vi "Vm_and_g1g2g3_Wrapper.vi"(0 "Path Array":string[](array[string])=["C:\\CuspControl\\GPIB and Network\\RGSBias.txt", "6723"], 1 "Input Values":dbl[](array[numeric])=[88.0, 1.0, 2.0, 3.0]) -> ()   [LabVIEW 2018]
uses:
  <vilib>/Analysis/1siggen.llb/Ramp Pattern by Samples.vi
  <vilib>/DAQmx/write.llb/DAQmx Write (Analog 1D DBL 1Chan NSamp).vi
  <vilib>/DAQmx/create/channels.llb/DAQmx Create Channel (AO-Voltage-Basic).vi
  <vilib>/DAQmx/configure/timing.llb/DAQmx Timing (Sample Clock).vi
  <vilib>/DAQmx/miscellaneous.llb/DAQmx Fill In Error Info.vi
  <vilib>/Analysis/NI_AALBase.lvlib
panel:
  out "Vout, gain, offset":dbl[][](array[numeric])=[[0.0, 161.0, -0.006], [70.5, 161.0, -0.006], [79.5, 161.0, -0.006], [83.0, 161.0, -0.006], [0.0, 0.0, 0.0], [0.0, 0.0, 0.0], [0.0, 0.0, 0.0], [0.0, 0.0, 0.0], [0.0, 0.0, 0.0]]
  out "Output Values":dbl[](array[numeric])=[88.0, 1.0, 2.0, 3.0]
  out "pathName":path=path "C:/CuspControl/GPIB and Network/RGSBias.txt"
  in  "rate":dbl=1000.0 format="%0.2f"
  in  "samples":i32=128
  out "Start Values":dbl[](array[numeric])=[-3.7267080745341614e-05, 0.4378509316770186, 0.4937515527950311, 0.5154906832298136]
  out "End Values":dbl[](array[numeric])=[0.5465465838509317, 0.0061739130434782605, 0.012385093167701863, 0.018596273291925466]
  out "Enable":bool[](array[boolean])=[TRUE, TRUE, TRUE, TRUE]
  out "Time (s)":dbl=0.5339438999999402
  out "Device names":string[](array[string])=["Dev8/ao4", "Dev8/ao1", "Dev8/ao2", "Dev8/ao3"]
  out "error out":errorcluster
  # "RGS Bias Dev5/ao4"
  # "2021-07-27 EDH\nwtf Andi it's not dev5\nseems to be dev8\nin any case, is PXI 6723"
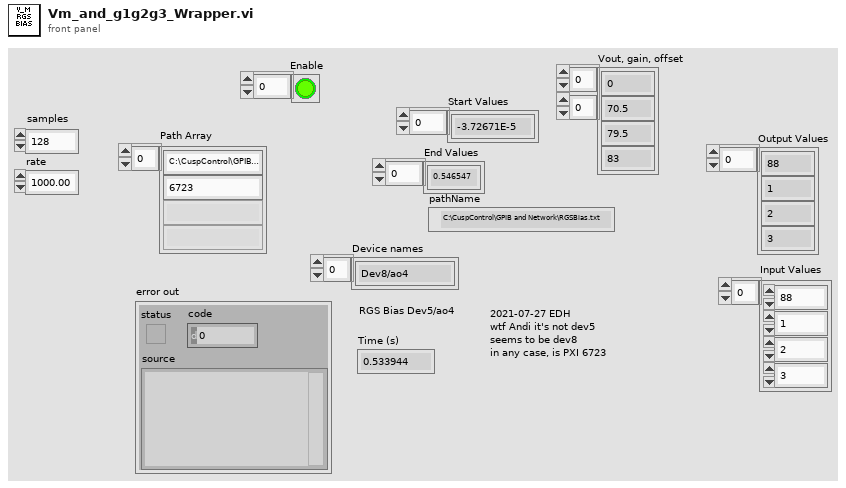
[diagram p1: front panel]
types:
  T1 = enum16{"open", "replace", "create", "open or create", "replace or create", "replace or create with confirmation"}
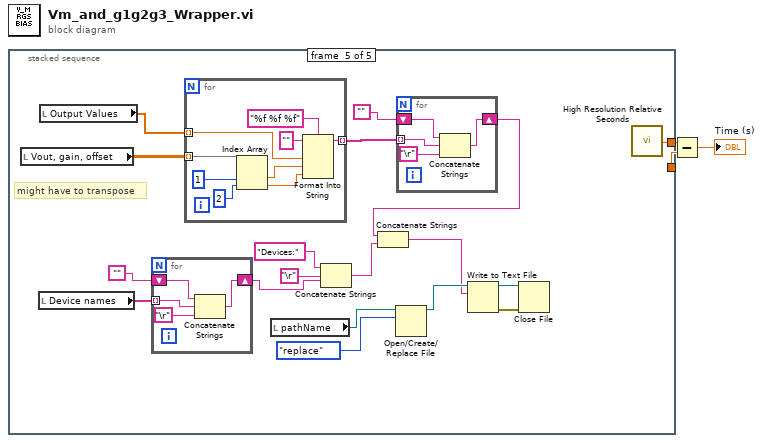
[diagram p0: block diagram]
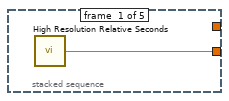
[diagram p2: hidden frame]
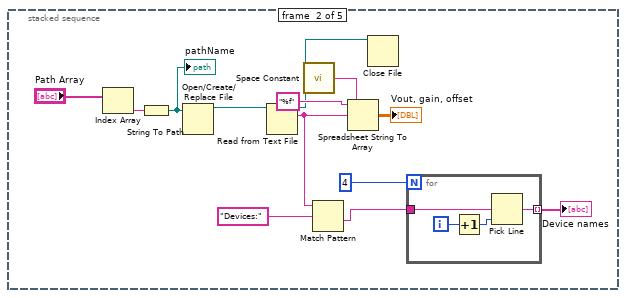
[diagram p3: hidden frame]
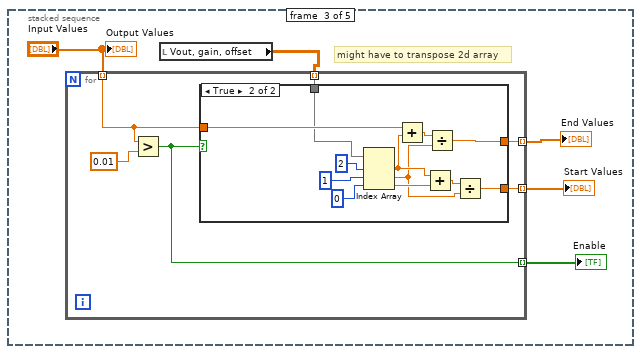
[diagram p4: hidden frame]
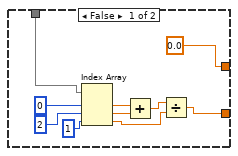
[diagram p5: hidden frame]
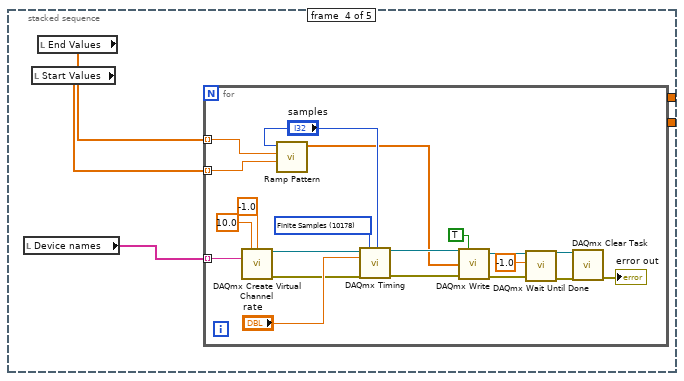
[diagram p6: hidden frame]
diagram:
  n1 = stacked-sequence {
    tunnel: [w4 _ _ _ _] -> w2
    tunnel: [_ _ _ _ w95] -> w3
    frame #0 {
      n2 = call <vilib>:"High Resolution Relative Seconds.vi"() -> ("relative seconds"=w4:dbl)
    }
    frame #1 {
      n3 = Index Array(array="Path Array") -> (element=w16:string)  [unwired: 1 in]
      n4 = String To Path(string=w16) -> (path=w7:path)
      "pathName" <- w7
      n5 = Open/Create/Replace File(file path (use dialog)=w7) -> (refnum out=w8:refnum<file>)  [unwired: 5 in, 2 out]
      n6 = Read from Text File(file (use dialog)=w8) -> (refnum out=w6:refnum<file>, text=w13:string)  [unwired: 3 in, 2 out]
      n7 = call <vilib>:"Space Constant.vi"() -> ("String"=w14:string)
      n8 = Match Pattern(string=w13, regular expression="Devices:") -> (after substring=w11:string)  [unwired: 1 in, 3 out]
      n9 = Spreadsheet String To Array(delimiter (Tab)=w14, format string="%f", spreadsheet string=w13) -> (array=→"Vout, gain, offset":dbl[][])  [unwired: 1 in]
      n10 = Close File(refnum=w6) -> ()  [unwired: 1 in, 2 out]
      n11 = for {
        N: 4 -> [_]
        tunnel: w11 -> [w19]
        tunnel: [w18] -> w9 mode=indexing
        i -> [w21]
        n12 = Increment(x=w21) -> (x+1=w20:i32)
        n13 = Pick Line(multi-line string=w19, line index=w20) -> (output string=w18:string)  [unwired: 1 in]
      }
      "Device names" <- w9
    }
    frame #2 {
      # "might have to transpose 2d array"
      n14 = local read "Vout, gain, offset"() -> (w22:dbl[][])
      n15 = for {
        tunnel: [w31] -> w26 mode=indexing
        tunnel: [w30] -> w25 mode=indexing
        tunnel: [w29] -> w24 mode=indexing
        tunnel: "Input Values" -> [w28] mode=indexing
        tunnel: w22 -> [w27] mode=indexing
        n16 = Greater?(x=w28, y=0.01) -> (0:w31:bool)
        n17 = case shown="True" w31 {
          tunnel: [0.0 w51] -> w30
          tunnel: w28 -> [_ w50]
          tunnel: [w39 w47] -> w29
          tunnel: w27 -> [w33 w43]
          frame False {
            n18 = Index Array(array=w33, index #1=0 ("index"), index #2=2 ("index"), index #3=1 ("index")) -> (element #1=w36:dbl, element #2=w35:dbl, element #3=w34:dbl)
            n19 = Add(x=w36, y=w35) -> (x+y=w41:dbl)
            n20 = Divide(x=w41, y=w34) -> (x/y=w39:dbl)
          }
          frame True {
            n21 = Index Array(array=w43, index #1=2 ("index"), index #2=1 ("index"), index #3=0 ("index")) -> (element #1=w45:dbl, element #2=w44:dbl, element #3=w46:dbl)
            n22 = Add(x=w50, y=w45) -> (x+y=w54:dbl)
            n23 = Add(x=w45, y=w46) -> (x+y=w48:dbl)
            n24 = Divide(x=w54, y=w44) -> (x/y=w51:dbl)
            n25 = Divide(x=w48, y=w44) -> (x/y=w47:dbl)
          }
        }
      }
      "Enable" <- w26
      "End Values" <- w25
      "Start Values" <- w24
      "Output Values" <- "Input Values"
    }
    frame #3 {
      n26 = local read "Device names"() -> (w55:string[])
      n27 = local read "Start Values"() -> (w56:dbl[])
      n28 = local read "End Values"() -> (w57:dbl[])
      n29 = for {
        tunnel: w57 -> [w74] mode=indexing
        tunnel: w56 -> [w73] mode=indexing
        tunnel: w55 -> [w58] mode=indexing
        w67 = 10178 items=["Finite Samples"=10178, "Continuous Samples"=10123, "Hardware Timed Single Point"=12522] ("sample mode")
        n30 = call-poly <vilib>:"DAQmx Create Virtual Channel.vi"("maximum value"=10.0, "minimum value"=-1.0, "physical channels"=w58) -> ("task out"=w72:refnum<k21>, "error out"=w70:errorcluster)  [unwired: 11 in]
        n31 = call-poly <vilib>:"Ramp Pattern.vi"("start"=w73, "end"=w74, "samples"="samples") -> ("Ramp Pattern"=w65:dbl[])  [unwired: 7 in, 1 out]
        n32 = call-poly <vilib>:"DAQmx Timing.vi"("task/channels in"=w72, "sample mode"=w67, "samples per channel"="samples", "rate"="rate", "error in"=w70) -> ("task out"=w69:refnum<k21>, "error out"=w68:errorcluster)  [unwired: 9 in]
        n33 = call-poly <vilib>:"DAQmx Write.vi"("task/channels in"=w69, "auto start"=TRUE, "data"=w65, "error in"=w68) -> ("task out"=w61:refnum<k21>, "error out"=w60:errorcluster)  [unwired: 9 in, 1 out]
        n34 = call <vilib>:"DAQmx Wait Until Done.vi"("task/channels in"=w61, "timeout (sec)"=-1.0, "error in"=w60) -> ("task out"=w62:refnum<k21>, "error out"=w63:errorcluster)  [unwired: 11 in]
        n35 = call <vilib>:"DAQmx Clear Task.vi"("task in"=w62, "error in"=w63) -> ("error out"=→"error out":errorcluster)  [unwired: 13 in]
      }
    }
    frame #4 {
      # "might have to transpose"
      n36 = local read "Vout, gain, offset"() -> (w81:dbl[][])
      n37 = local read "Device names"() -> (w84:string[])
      n38 = local read "Output Values"() -> (w85:dbl[])
      n39 = for {
        tunnel: w84 -> [w102] mode=indexing
        shift-right: [w101] -> w83
        shift-left: "" -> [w100]
        n40 = Concatenate Strings(w100, w102, "\r") -> (w101:string)
      }
      n41 = for {
        tunnel: w81 -> [w111] mode=indexing
        tunnel: [w105] -> w79 mode=indexing
        tunnel: w85 -> [w104] mode=indexing
        n42 = Index Array(array=w111, index #1=1 ("index"), index #2=2 ("index")) -> (element #1=w108:dbl, element #2=w107:dbl)
        n43 = Format Into String(format string="%f %f %f", initial string="", w104, w108, w107) -> (resulting string=w105:string)  [unwired: 1 in, 1 out]
      }
      n44 = local read "pathName"() -> (w91:path)
      n45 = Concatenate Strings("Devices:" ("string"), "\r", w83) -> (w94:string)
      n46 = Open/Create/Replace File(file path (use dialog)=w91, operation (0:open)=T1."replace") -> (refnum out=w89:refnum<file>)  [unwired: 4 in, 2 out]
      n47 = for {
        tunnel: w79 -> [w98] mode=indexing
        shift-right: [w96] -> w78
        shift-left: "" -> [w97]
        n48 = Concatenate Strings(w97, w98, "\r") -> (w96:string)
      }
      n49 = Concatenate Strings(w78, w94) -> (w88:string)
      n50 = Write to Text File(file (use dialog)=w89, text=w88) -> (refnum out=w86:refnum<file>, error out=w87:errorcluster)  [unwired: 2 in, 1 out]
      n51 = Close File(refnum=w86, error in=w87) -> ()  [unwired: 2 out]
      n52 = call <vilib>:"High Resolution Relative Seconds.vi"() -> ("relative seconds"=w95:dbl)
    }
  }
  n53 = Subtract(x=w3, y=w2) -> (x-y=→"Time (s)":dbl)
